vi "modbus test.vi"() -> ()   [LabVIEW 2019]
uses:
  <vilib>/Platform/TimedLoop/XDataNode/timing_clust.ctl
  <vilib>/Platform/TimedLoop/XDataNode/nitl_modes.ctl
  <vilib>/Platform/TimedLoop/XDataNode/wakeup.ctl
  <vilib>/NI/Modbus Library/API/Wrapper/Create TCP Slave.vi
  <vilib>/platform/TimedLoop/XDataNode/XDataNode.xnode
  <vilib>/NI/Modbus Library/API/Slave/Modbus Slave.lvclass
  <vilib>/NI/Modbus Library/API/Wrapper/API Main.lvlib
  <vilib>/Platform/TimedLoop/XDataNode/XDNodeRunTimeDep.lvlib
panel:
  out "size(s)":i32
  out "coils":bool[](array[boolean])
  out "register values":u16[](array[numeric])
  in  "coils to write":bool[](array[boolean])
  in  "registers to write":u16[](array[numeric])
  in  "Cluster":T1
  in  "Period":i64=1
  out "error out":errorcluster
  in  "write starting address":u16
  out "real period":u32
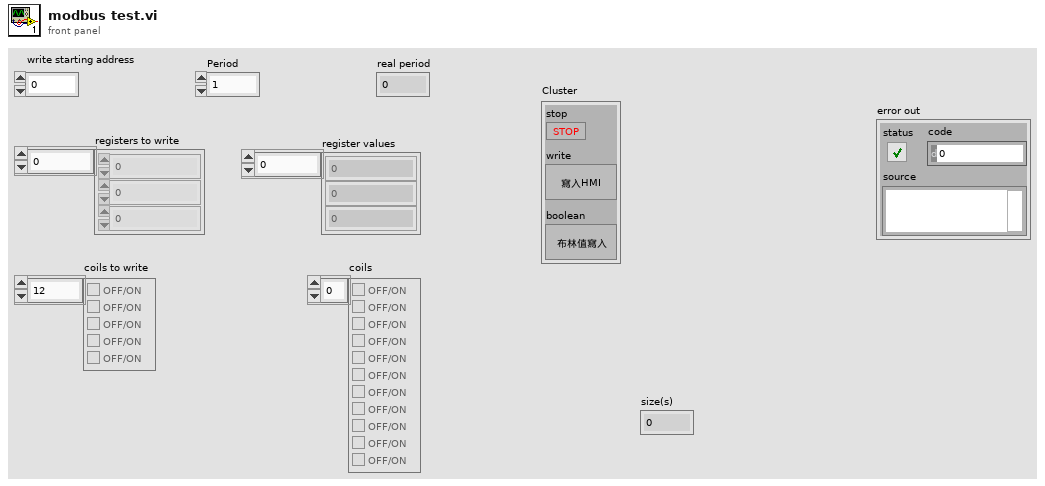
[diagram p1: front panel]
types:
  T1 = cluster{"stop":bool, "write":bool, "boolean":bool}
  T2 = typedef "XDNodeRunTimeDep.lvlib/timing_clust.ctl" = cluster{"Expected End [f-1]":u64, "Actual End [f-1]":u64, "Finished Late? [f-1]":bool, "Expected End [i-1]":u64, "Actual End [i-1]":u64, "Finished Late? [i-1]":bool, "Expected Start [i]":u64, "Actual Start [i]":u64, "Expected Start [f]":u64, "Actual Start [f]":u64, "Source Name":string, "Structure Name":string, "Period":i64, "Deadline":i64, "Offset":i64, "Start":i64, "Priority":i32, "Timeout":i32, "Mode":T3, "Wakeup Reason":T4, "Error":errorcluster, "Source Type":string, "Secondary Source Type":string, "Global End Time":u64, "Global Start Time":u64, "Frame Duration":u64, "Iteration Duration":u64, "Assigned CPU":i32, "I/O Scan Engine Mode":u32}
  T3 = typedef "XDNodeRunTimeDep.lvlib/nitl_modes.ctl" = enum32{"No Change", "Process missed periods, maintain original phase", "Discard missed periods, maintain original phase", "Process missed periods, ignore original phase", "Discard missed periods, ignore original phase"}
  T4 = typedef "XDNodeRunTimeDep.lvlib/wakeup.ctl" = enum32{"Normal", "Aborted", "Asynchronous wakeup", "Timing source error", "Timed loop error", "Timeout"}
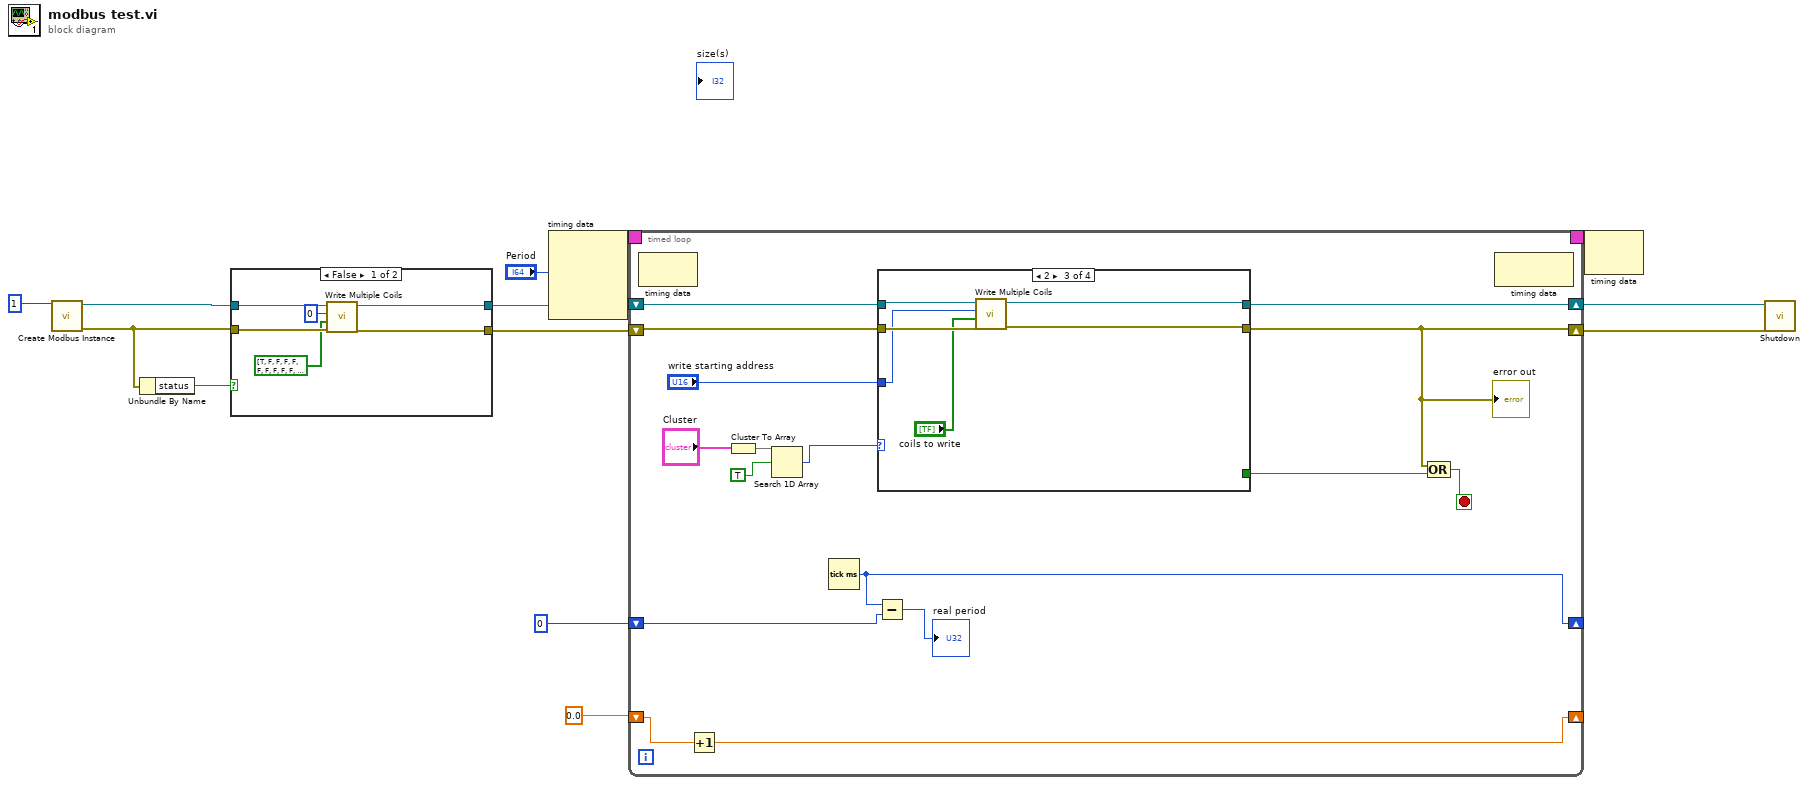
[diagram p0: block diagram]
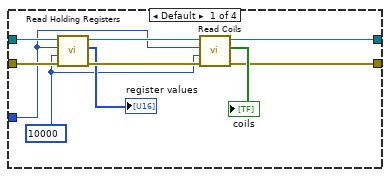
[diagram p2: hidden frame]
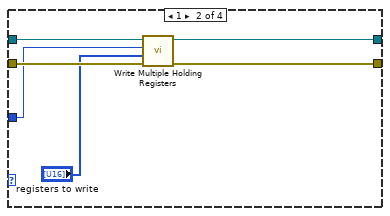
[diagram p3: hidden frame]
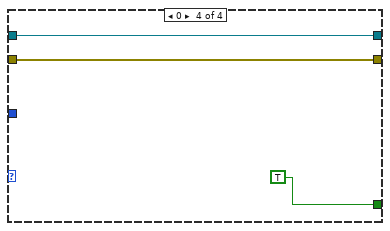
[diagram p4: hidden frame]
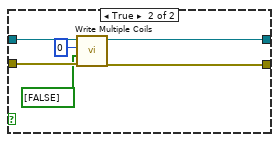
[diagram p5: hidden frame]
diagram:
  n1 = call-poly <vilib>:"Create Modbus Instance.vi"("port (502)"=u16 1) -> ("error out"=w6:errorcluster, "TCP slave instance"=w7:refnum<class "Modbus Slave.lvclass">)  [unwired: 9 in]
  n2 = Unbundle By Name(w6) -> ("status"=w8:bool)
  n3 = case shown="False" w8 {
    tunnel: w7 -> [w19 w25]
    tunnel: w6 -> [w18 w24]
    tunnel: [w17 w22] -> w4
    tunnel: [w16 w21] -> w3
    frame False {
      n4 = call-dynamic "Write Multiple Coils.vi"("error in"=w18, "coils to write"=bool[] [TRUE, FALSE, FALSE, FALSE, FALSE, FALSE, FALSE, FALSE, FALSE, FALSE, FALSE, FALSE, FALSE, FALSE, FALSE, FALSE, FALSE, FALSE, FALSE, FALSE, FALSE, FALSE, FALSE, FALSE, FALSE, FALSE, FALSE, FALSE, FALSE, FALSE, FALSE, FALSE, FALSE, FALSE, FALSE, FALSE, FALSE, FALSE, FALSE, FALSE, FALSE, FALSE, FALSE, FALSE, FALSE, FALSE, FALSE, FALSE, FALSE, FALSE, FALSE, FALSE, FALSE, FALSE, FALSE, FALSE, FALSE, FALSE, FALSE, FALSE, FALSE, FALSE, FALSE, FALSE, FALSE, FALSE, FALSE, FALSE, FALSE, FALSE, FALSE, FALSE, FALSE, FALSE, FALSE, FALSE, FALSE, FALSE, FALSE, FALSE, FALSE, FALSE, FALSE, FALSE, FALSE, FALSE, FALSE, FALSE, FALSE, FALSE, FALSE, FALSE, FALSE, FALSE, FALSE, FALSE, FALSE, FALSE, FALSE, TRUE], "starting address"=u16 0, "Modbus slave in"=w19) -> ("error out"=w16:errorcluster, "Modbus slave out"=w17:refnum<class "Modbus Slave.lvclass">)  [unwired: 6 in]
    }
    frame True {
      n5 = call-dynamic "Write Multiple Coils.vi"("error in"=w24, "coils to write"=bool[] [FALSE], "starting address"=u16 0, "Modbus slave in"=w25) -> ("error out"=w21:errorcluster, "Modbus slave out"=w22:refnum<class "Modbus Slave.lvclass">)  [unwired: 6 in]
    }
  }
  n6 = node-c288("Period") -> (w13:T2)  [unwired: 3 in]
  n7 = timed-loop {
    shift-right: [w29] -> w10
    shift-left: w3 -> [w32]
    shift-right: [w31] -> w11
    shift-left: w4 -> [w33]
    timing: w13 -> [_]
    timing-out: [_] -> w12
    shift-right: [w38] -> _
    shift-left: u32 0 ("millisecond timer value") -> [w39]
    shift-right: [w26] -> _
    shift-left: 0.0 -> [w27]
    stop <- w41 stop-if-true
    n8 = node-c288() -> ()  [unwired: 1 in, 1 out]
    n9 = Increment(x=w27) -> (x+1=w26:dbl)
    n10 = Cluster To Array(cluster="Cluster") -> (array=w36:bool[])
    n11 = Search 1D Array(1D array=w36, element=TRUE) -> (index of element=w34:i32)  [unwired: 1 in]
    n12 = Tick Count (ms)() -> (millisecond timer value=w38:u32)
    n13 = Subtract(x=w38, y=w39) -> (x-y=→"real period":u32)
    n14 = case shown="2" w34 {
      tunnel: w33 -> [w51 w57 w63 w65]
      tunnel: w32 -> [w50 w56 w62 w64]
      tunnel: [w42 w54 w59 w65] -> w31
      tunnel: [w43 w53 w58 w64] -> w29
      tunnel: "write starting address" -> [w44 w55 w61 _]
      tunnel: [_ _ _ TRUE] -> w28
      frame Default {
        w45 = u16 10000 ("number of inputs")
        n15 = call-dynamic "Read Holding Registers.vi"("error in"=w50, "number of inputs"=w45, "starting address"=w44, "Modbus slave in"=w51) -> ("error out"=w48:errorcluster, "register values"=→"register values":u16[], "Modbus slave out"=w49:refnum<class "Modbus Slave.lvclass">)  [unwired: 5 in]
        n16 = call-dynamic "Read Coils.vi"("error in"=w48, "number of inputs"=w45, "starting address"=w44, "Modbus slave in"=w49) -> ("error out"=w43:errorcluster, "coils"=→"coils":bool[], "Modbus slave out"=w42:refnum<class "Modbus Slave.lvclass">)  [unwired: 5 in]
      }
      frame 1 {
        n17 = call-dynamic "Write Multiple Holding Registers.vi"("error in"=w56, "registers to write"="registers to write", "starting address"=w55, "Modbus slave in"=w57) -> ("error out"=w53:errorcluster, "Modbus slave out"=w54:refnum<class "Modbus Slave.lvclass">)  [unwired: 6 in]
      }
      frame 2 {
        n18 = call-dynamic "Write Multiple Coils.vi"("error in"=w62, "coils to write"="coils to write", "starting address"=w61, "Modbus slave in"=w63) -> ("error out"=w58:errorcluster, "Modbus slave out"=w59:refnum<class "Modbus Slave.lvclass">)  [unwired: 6 in]
      }
      frame 0 {
      }
    }
    "error out" <- w29
    n19 = Compound Arithmetic op=OR(w29, w28) -> (w41:bool)
    n20 = node-c288() -> ()  [unwired: 1 in, 1 out]
  }
  n21 = node-c288(w12) -> ()  [unwired: 1 out]
  n22 = call-dynamic "Shutdown.vi"("error in"=w10, "Modbus slave in"=w11) -> ()  [unwired: 9 in, 1 out]
